vi "Input leakage currents and offset voltage.vi"(0 "数组输入":dbl[](array[numeric])) -> (4 "Voffset":dbl, 6 "Iin-":dbl, 8 "Iin+":dbl, 10 "Iin_mean":dbl, 15 "Iin_bias":dbl)   [LabVIEW 2019]
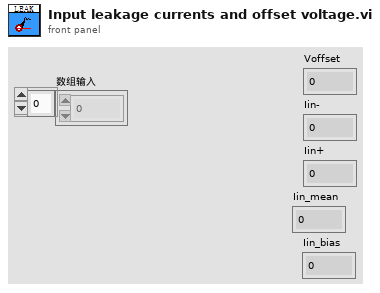
[diagram p1: front panel]
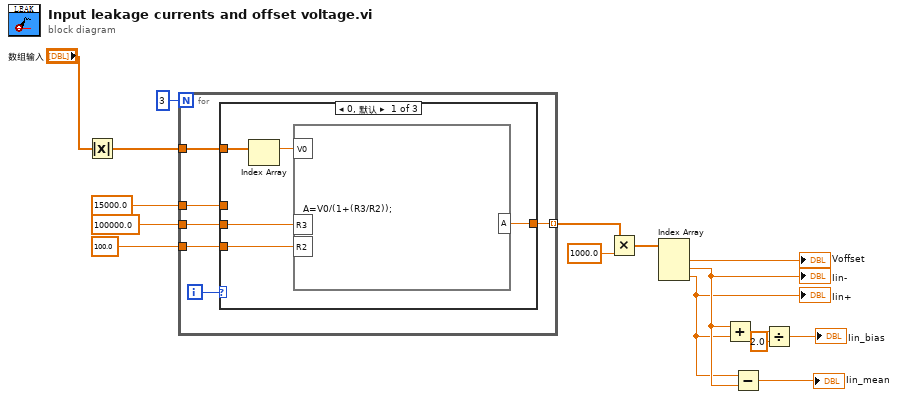
[diagram p0: block diagram]
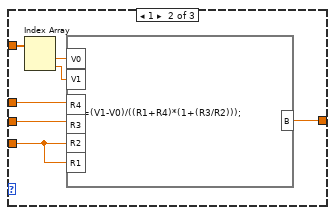
[diagram p2: hidden frame]
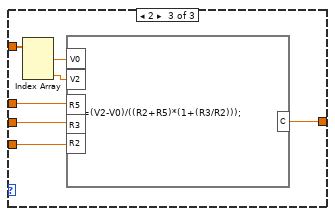
[diagram p3: hidden frame]
diagram:
  n1 = Absolute Value(x="数组输入") -> (abs(x)=w8:dbl[])
  n2 = for {
    N: 3 -> [_]
    tunnel: w8 -> [w21]
    tunnel: 100.0 ("输入变量") -> [w20]
    tunnel: 100000.0 ("输入变量") -> [w19]
    tunnel: [w18] -> w16 mode=indexing
    tunnel: 15000.0 ("输入变量") -> [w17]
    i -> [w22]
    n3 = case shown="0, 默认" w22 {
      tunnel: w21 -> [w25 w31 w37]
      tunnel: w20 -> [w27 w28 w41]
      tunnel: w19 -> [w26 w34 w40]
      tunnel: [w23 w33 w39] -> w18
      tunnel: w17 -> [_ w32 w38]
      frame 0, Default {
        n4 = Index Array(array=w25) -> (element=w24:dbl)  [unwired: 1 in]
        n5 = formula code="A=V0/(1+(R3/R2));"("R3"=w26, "R2"=w27, "V0"=w24) -> ("A"=w23:dbl)
      }
      frame 1 {
        n6 = Index Array(array=w31) -> (element #1=w30:dbl, element #2=w29:dbl)  [unwired: 2 in]
        n7 = formula code="B=(V1-V0)/((R1+R4)*(1+(R3/R2)));"("R3"=w34, "R2"=w28, "V0"=w30, "R1"=w28, "R4"=w32, "V1"=w29) -> ("B"=w33:dbl)
      }
      frame 2 {
        n8 = Index Array(array=w37) -> (element #1=w36:dbl, element #3=w35:dbl)  [unwired: 3 in, 1 out]
        n9 = formula code="C=(V2-V0)/((R2+R5)*(1+(R3/R2)));"("R3"=w40, "R2"=w41, "V0"=w36, "R5"=w38, "V2"=w35) -> ("C"=w39:dbl)
      }
    }
  }
  n10 = Multiply(x=w16, y=1000.0) -> (x*y=w4:dbl[])
  n11 = Index Array(array=w4) -> (element #1=→"Voffset":dbl, element #2=w6:dbl, element #3=w5:dbl)  [unwired: 3 in]
  "Iin-" <- w6
  "Iin+" <- w5
  n12 = Add(x=w6, y=w5) -> (x+y=w14:dbl)
  n13 = Subtract(x=w5, y=w6) -> (x-y=→"Iin_mean":dbl)
  n14 = Divide(x=w14, y=2.0) -> (x/y=→"Iin_bias":dbl)
